vi "3Act Helper - SailSettingToDynamixelDegrees.vi"(10 "SailSuggestion":dbl, 11 "Dynamixel Set Data":T1) -> (3 "Dynamixel Angle":dbl)   [LabVIEW 2013]
doc: "This VI takes in a 0-1 sail setting and turns it into degree values for the Dynamixel. This is based strongly on the upper and lower bounds for the Dynamixel, which should be set from the OCU.\n\nEric Schneider, March 2014"
uses:
  Data/TypeDefs/DynamixelSetupInfo.ctl
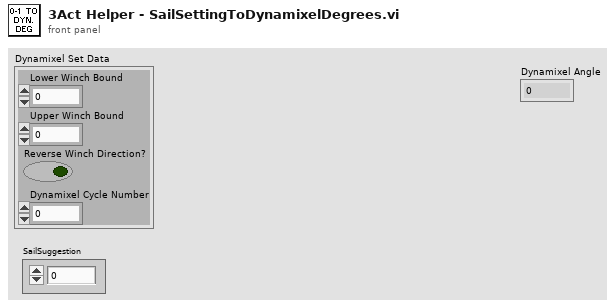
[diagram p1: front panel]
types:
  T1 = typedef "DynamixelSetupInfo.ctl" = cluster{"Lower Winch Bound":dbl, "Upper Winch Bound":dbl, "Reverse Winch Direction?":bool, "Dynamixel Cycle Number":i32}
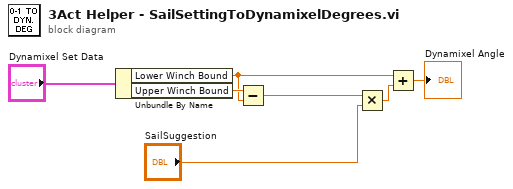
[diagram p0: block diagram]
diagram:
  n1 = Unbundle By Name("Dynamixel Set Data") -> ("Lower Winch Bound"=w5:dbl, "Upper Winch Bound"=w6:dbl)
  n2 = Subtract(x=w6, y=w5) -> (x-y=w3:dbl)
  n3 = Multiply(x=w3, y="SailSuggestion") -> (x*y=w2:dbl)
  n4 = Add(x=w5, y=w2) -> (x+y=→"Dynamixel Angle":dbl)
